vi "Get SA by Address.vi"(8 "error in":errorcluster, 10 "address":i8, 11 "remote terminal ref in":refnum<k24>) -> (0 "error out":errorcluster, 1 "remote terminal":refnum<k24>, 2 "found":bool, 3 "remote terminal ref out":refnum<k24>)   [LabVIEW 2020, in "Ballard_1553_Hardware_ni.lvlib"]
uses:
  Ballard_1553_Hardware_ni.lvlib
  C:/Users/Administrator/Desktop/GIT/Ballard-MIL-STD-1553-Custom-Device/Source/System Explorer/SubVIs/Parse XML Ballard/1.2/BTIXML_SerDes.dll
  Ballard-MIL-STD-1553-Custom-Device/Source/System Explorer/SubVIs/Parse XML Ballard/1.2/BTIXML_SerDes.dll
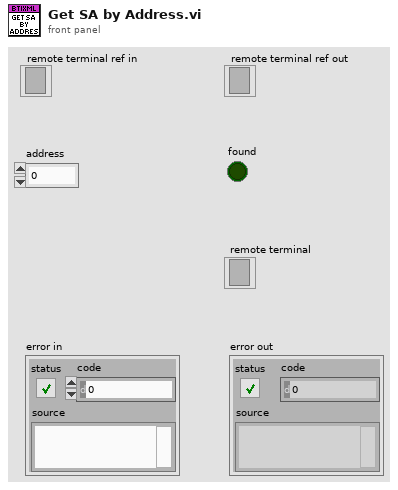
[diagram p1: front panel]
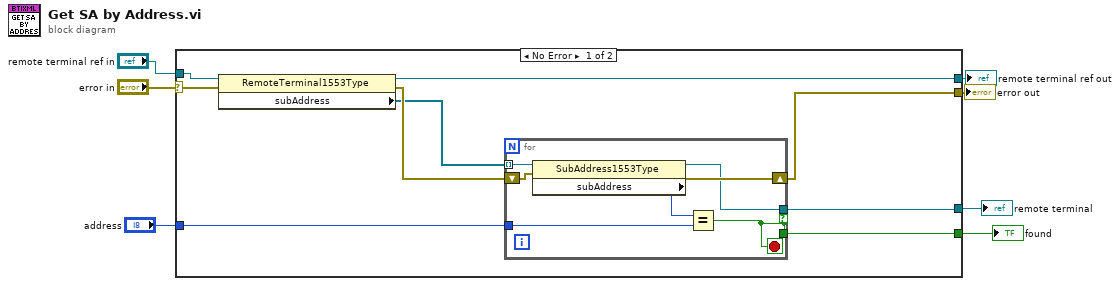
[diagram p0: block diagram]
diagram:
  n1 = case shown="No Error" "error in" {
    selector: "error in" -> [w13 w24]
    tunnel: [w10 w24] -> w7
    tunnel: [w16 w25] -> w6
    tunnel: "remote terminal ref in" -> [w15 w25]
    tunnel: "address" -> [w12 _]
    tunnel: [w11 _] -> w2
    tunnel: [w9 _] -> w1
    frame No Error {
      n2 = property class="RemoteTerminal1553Type"(reference=w15, error in=w13) -> (reference out=w16:refnum<k24>, error out=w14:errorcluster, "subAddress"=w8:refnum<k24>[])
      n3 = for {
        shift-right: [w19] -> w10
        shift-left: w14 -> [w22]
        tunnel: w12 -> [w20]
        tunnel: w8 -> [w23] mode=indexing
        tunnel: [w18] -> w9 if=w17
        tunnel: [w17] -> w11
        stop <- w17 stop-if-true
        n4 = property class="SubAddress1553Type"(reference=w23, error in=w22) -> (reference out=w18:refnum<k24>, error out=w19:errorcluster, "subAddress"=w21:i8)
        n5 = Equal?(x=w21, y=w20) -> (x = y?=w17:bool)
      }
    }
    frame Error {
    }
  }
  "error out" <- w7
  "remote terminal ref out" <- w6
  "remote terminal" <- w1
  "found" <- w2
